vi "Average_Image_in_y-Direction.vi"(8 "Cut image":dbl[][](array[numeric])) -> (1 "X-Axis":dbl[](array[numeric]), 2 "Intensity Average":dbl[](array[numeric]))   [LabVIEW 2014]
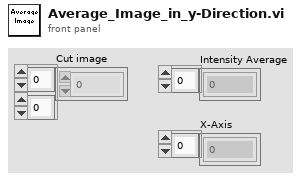
[diagram p1: front panel]
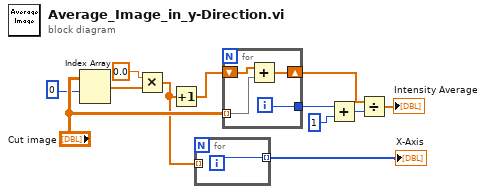
[diagram p0: block diagram]
diagram:
  n1 = Index Array(array="Cut image", index (row)=u32 0 ("Active Cursor")) -> (element=w2:dbl[])  [unwired: 1 in]
  n2 = Multiply(x=0.0 ("element"), y=w2) -> (x*y=w1:dbl[])
  n3 = Increment(x=w1) -> (x+1=w8:dbl[])
  n4 = for {
    tunnel: w1 -> [_] mode=indexing
    tunnel: [w13] -> w10 mode=indexing
    i -> [w13]
  }
  "X-Axis" <- w10
  n5 = for {
    tunnel: "Cut image" -> [w16] mode=indexing
    shift-right: [w15] -> w9
    shift-left: w8 -> [w17]
    tunnel: [w14] -> w5
    i -> [w14]
    n6 = Add(x=w17, y=w16) -> (x+y=w15:dbl[])
  }
  n7 = Add(x=w5, y=u32 1 ("Active Cursor")) -> (x+y=w7:u32)
  n8 = Divide(x=w9, y=w7) -> (x/y=→"Intensity Average":dbl[])
